vi "Ex1_StateMachines.vi"() -> ()   [LabVIEW 2024]
uses:
  Control 1.ctl
panel:
  out "Waveform Chart":dbl(graph)
  in  "Threshold":dbl
  in  "Measure Button":bool
  in  "Add to chart Button":bool
  out "Measured Value":dbl
  in  "STOP":bool
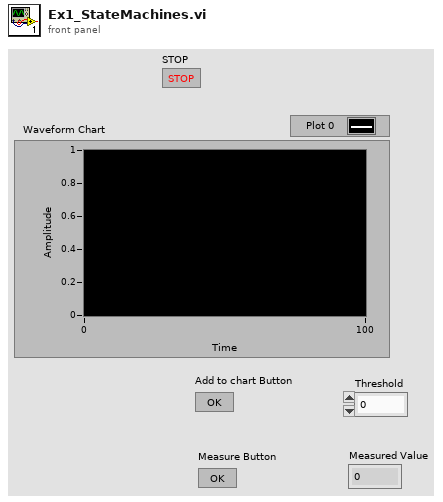
[diagram p1: front panel]
types:
  T1 = typedef "Control 1.ctl" = enum16{"Idle", "Add to chart", "Measure"}
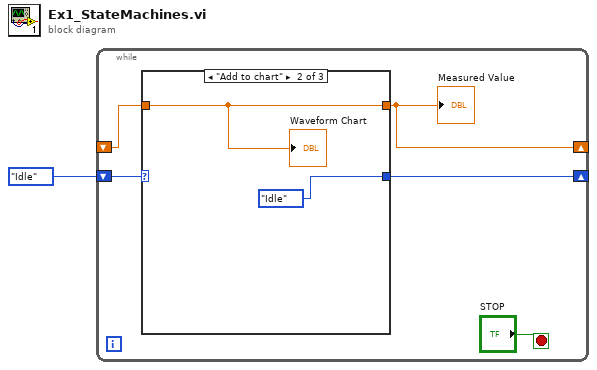
[diagram p0: block diagram]
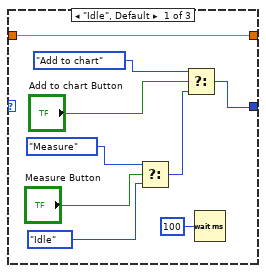
[diagram p2: hidden frame]
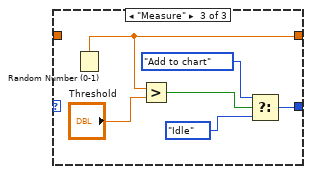
[diagram p3: hidden frame]
diagram:
  n1 = while {
    shift-right: [w5] -> _
    shift-left: _ -> [w4]
    shift-right: [w3] -> _
    shift-left: Control_1."Idle" -> [w2]
    stop <- "STOP" stop-if-true
    n2 = case shown="\"Add to chart\"" w2 {
      tunnel: [w15 w17 w22] -> w5
      tunnel: w4 -> [w15 w17 _]
      tunnel: [w9 Control_1."Idle" w21] -> w3
      frame "Idle", Default {
        n3 = Select(t=Control_1."Measure", s="Measure Button", f=Control_1."Idle") -> (s? t:f=w11:T1)
        n4 = Select(t=Control_1."Add to chart", s="Add to chart Button", f=w11) -> (s? t:f=w9:T1)
        n5 = Wait (ms)(milliseconds to wait=100) -> ()  [unwired: 1 out]
      }
      frame "Add to chart" {
        "Waveform Chart" <- w17
      }
      frame "Measure" {
        n6 = Random Number (0-1)() -> (number: 0 to 1=w22:dbl)
        n7 = Greater?(x=w22, y="Threshold") -> (0:w19:bool)
        n8 = Select(t=Control_1."Add to chart", s=w19, f=Control_1."Idle") -> (s? t:f=w21:T1)
      }
    }
    "Measured Value" <- w5
  }
